vi "AlliGator Script Sequential ROIs Time-Gated Data Series NLSF Analysis.vi"(4 "AlliGator Data Series Type":T10, 8 "Error In":errorcluster, 9 "AlliGator Ctrl Refnums":T1, 10 "Path":path, 11 "Alligator Queue Elements in":T11[](array[typedef])) -> (0 "Error Out":errorcluster, 1 "Message":string, 2 "Time-Series Paths":path[](array[path]), 3 "Alligator Queue Elements out":T11[](array[typedef]))   [LabVIEW 2021, in "AlliGator Scripts.lvlib"]
doc: "Script performing NLSF analysis of a different ROI for each dataset in a series. This is used for instance if the ROI list is representing the successive locations of an object being tracked across the dataset series."
uses:
  AlliGator Scripts.lvlib
  Action Engine/AlliGator Q Element.ctl
  Action Engine/AlliGator Q Event.ctl
  Files/AlliGator Data Series Type.ctl
  GUI/AlliGator Ctrl Refnums.ctl
  GUI/AlliGator Other Ctrl Refnums.ctl
  GUI/AlliGator State Indicator.ctl
  GUI/AlliGator Main Window Tabs.ctl
  GUI/AlliGator Phasor Plot Ctrl Refnums.ctl
  GUI/AlliGator Phasor Graph Ctrl Refnums.ctl
  Phasor/Phasor Calibration Type.ctl
  GUI/AlliGator Dataset Ctrl Refnums.ctl
  Source Image/AlliGator Displayed Image.ctl
  GUI/AlliGator Registered Events Ctrl Refnums.ctl
  GUI/AlliGator Image Histogram Control Refnums.ctl
  Histograms/Linear Histogram Options.ctl
  Histograms/Histogram Bin Option.ctl
  Histograms/Histogram Bin Position.ctl
  Decay Fit Parameter Map/AlliGator Decay Fit Map Control Refnums.ctl
  Fits/IRF(X)PSED/Decay Fit Parameters & Derived Quantities List v2.ctl
  Parameter Map/AlliGator Parameter Map Control Refnums.ctl
  Globals, Variables, Constants/AlliGator Variables List.ctl
  Action Engine/Alligator Elements Order in Action Stack.ctl
  Settings/AlliGator Settings List.ctl
  Fits/Decay Convolution/Decay Model.ctl
  Fits/Residual Type.ctl
  Fits/Non-linear Fitting Method v2.ctl
  Fits/Fit Calculation Method.ctl
  Fits/Non-linear Fitting Algorithm.ctl
  Graphs/XY Graph/New Plot Information.ctl
  Graphs/Plot Scales.ctl
  Graphs/LabVIEW Plot Interpolation.ctl
  Graphs/Plot Point Style.ctl
  ROIs/AlliGator ROI Manager Actions.ctl
  ROIs/AlliGator ROI Selection Data.ctl
  Graphs/XY Graph/XY Graph Selected Plot Info+Flag.ctl
  Graphs/XY Graph/XY Graph Refnum.ctl
  <vilib>/Utility/miscctls.llb/LVPoint32TypeDef.ctl
  Files/AlliGator FLI Dataset Type.ctl
  Action Engine/AlliGator Add Action Array to Stack.vi
  Action Engine/AlliGator Add Single Action to Stack.vi
  Action Engine/AlliGator Action Engine.lvlib
  Globals, Variables, Constants/AlliGator Globals, Variables & Constants.lvlib
  Decay Analysis/Decay Fit/AlliGator Decay Fit.lvlib
  Settings/AlliGator Settings.lvlib
  Fits/Fits.lvlib
  Strings/Strings.lvlib
  Files/Files.lvlib
  Files/AlliGator Files.lvlib
  Graphs/XY Graph/XY Graph Add-Ons.lvlib
  Graphs/Graphs.lvlib
  Variant/Variant.lvlib
  ROIs/AlliGator ROIs.lvlib
  Fits/IRF(X)PSED/Fit Weights Type v2.ctl
  Fits/IRF(X)PSED/Decay Fit Options v4.ctl
  Source Image/AlliGator Source Image.lvlib
  GUI/AlliGator GUI.lvlib
  Phasor/Phasor.lvlib
  Histograms/Histogram Window.lvlib
  Decay Fit Parameter Map/AlliGator Decay Fit Parameter Map.lvlib
  Parameter Map/AlliGator Parameter Map.lvlib
panel:
  out "# Time Points":i32
  # "see the AlliGator License on the block diagram (Ctrl+E or Window:Show Block Diagram)"
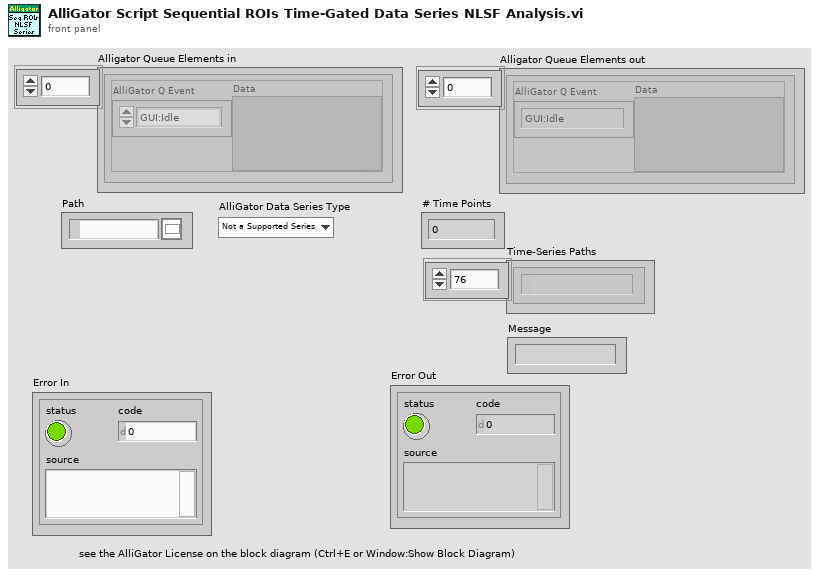
[diagram p1: front panel]
types:
  T1 = typedef "AlliGator GUI.lvlib/AlliGator Ctrl Refnums.ctl" = cluster{"Other AlliGator Ctrl Refnums":T2, "Phasor Plot Ctrl Refnums":T3, "Phasor Graph Ctrl Refnums":T4, "Dataset Control Refnums":T5, "Registered Events Ctrl Refnums":T6, "Image Histogram Ctrl Refnums":T7, "Decay Fit Map Ctrl Refnums":T8, "Parameter Map Ctrl Refnums":T9}
  T2 = typedef "AlliGator GUI.lvlib/AlliGator Other Ctrl Refnums.ctl" = cluster{"State Indicators":refnum<vi>, " Progress Bar":refnum<vi>, "Decay Graph Active":refnum<vi>, "Decay Statistics Bin":refnum<vi>, "Time Step":refnum<vi>, "Use File Timestamp":refnum<vi>, "Tab Control":refnum<vi>, "CPU":refnum<vi>, "Abort Fit":refnum<vi>, "Dataset File/Folder Path":refnum<vi>, "Abort ROI Creation":refnum<vi>, "Event LED":refnum<vi>, "Dataset File/Folder Path 2":refnum<vi>, "Dataset File/Folder Path 3":refnum<vi>, "Dataset File/Folder Path 4":refnum<vi>, "Dataset File/Folder Path 5":refnum<vi>, "Dataset File/Folder Path 6":refnum<vi>, "Dataset File/Folder Path 7":refnum<vi>, "Dataset File/Folder Path 8":refnum<vi>, "Dataset File/Folder Path 9":refnum<vi>, "Dataset File/Folder Path 10":refnum<vi>, "Dataset File/Folder Path 11":refnum<vi>}
  T3 = typedef "AlliGator GUI.lvlib/AlliGator Phasor Plot Ctrl Refnums.ctl" = cluster{"Phasor Ratio":refnum<vi>, "Modulus Lifetime":refnum<vi>, "Phasor at cursor (m, phi)":refnum<vi>, "Phase Lifetime":refnum<vi>, "Phasor at cursor (g, s)":refnum<vi>, "Phasor Plor Average Lifetime":refnum<vi>, "Phasor Plot Active":refnum<vi>, "Save Phasor Plot":refnum<vi>, "Image Overlay Color":refnum<vi>, "Phasor Plot Color Scale":refnum<vi>, "Reference 1 Button":refnum<vi>, "Reference 2 Button":refnum<vi>, "True Phasor Plot Value":refnum<vi>}
  T4 = typedef "AlliGator GUI.lvlib/AlliGator Phasor Graph Ctrl Refnums.ctl" = cluster{"Phasor Ratio":refnum<vi>, "Modulus Lifetime":refnum<vi>, "Phasor at cursor (m, phi)":refnum<vi>, "Phase Lifetime":refnum<vi>, "Phasor at cursor (g, s)":refnum<vi>, "Phasor Graph Average Lifetime":refnum<vi>, "Phasor Graph Active":refnum<vi>, "Save Phasor Graph":refnum<vi>, "Phasor Frame Slide":refnum<vi>, "Single Step Phasor":refnum<vi>, "Calibration Type":refnum<vi>, "Show Line":refnum<vi>, "Phase Lifetime 1":refnum<vi>, "Phase Lifetime 2":refnum<vi>, "Phasor Graph Frequency":refnum<vi>, "Phasor Reference 1 Control":refnum<vi>, "Phasor Reference 2 Control":refnum<vi>, "Calibration Lifetime":refnum<vi>, "Phase Lifetime SDV":refnum<vi>, "Average Lifetime SDV":refnum<vi>, "Phasor Ratio SDV":refnum<vi>, "Modulus Lifetime SDV":refnum<vi>}
  T5 = typedef "AlliGator GUI.lvlib/AlliGator Dataset Ctrl Refnums.ctl" = cluster{"Current Data":refnum<vi>, "Gate Image Slide":refnum<vi>, "Time Point Slide":refnum<vi>, "Current Time Stamp":refnum<vi>, "Save Image":refnum<vi>, "Displayed Image":refnum<vi>, "Overlay Mode":refnum<vi>, "Phasor Overlay Color":refnum<vi>, "Image Color Scale":refnum<vi>, "Use ROI as Search Area":refnum<vi>, "Source Image ROI Color":refnum<vi>, "True Pixel Value":refnum<vi>}
  T6 = typedef "AlliGator GUI.lvlib/AlliGator Registered Events Ctrl Refnums.ctl" = cluster{"Time Point Slider":refnum<vi>, "Phasor Plot Display Range":refnum<vi>, "Decay Graph":refnum<vi>, "Decay Statistics Graph":refnum<vi>, "Intensity Time Trace":refnum<vi>, "Phasor Graph":refnum<vi>, "Phasor Ratio Graph":refnum<vi>, "Lifetime Graph":refnum<vi>, "Phasor Plot Display":refnum<vi>, "Source Image Display":refnum<vi>, "Decay Fit Parameter Map Display Range":refnum<vi>, "Decay Fit Parameter Map Display":refnum<vi>, "Parameter Map Display Range":refnum<vi>, "Parameter Map Display":refnum<vi>, "Phasor Plot Display Range":refnum<vi>}
  T7 = typedef "AlliGator GUI.lvlib/AlliGator Image Histogram Control Refnums.ctl" = cluster{"Image Histogram":refnum<vi>, "Image Histogram Options":refnum<vi>, "Image Histogram Active":refnum<vi>, "Image Histogram Upper Percentile":refnum<vi>, "Image Histogram Lower Percentile":refnum<vi>, "Auto-Adjust Contrast":refnum<vi>}
  T8 = typedef "AlliGator Decay Fit Parameter Map.lvlib/AlliGator Decay Fit Map Control Refnums.ctl" = cluster{"Decay Fit Parameter Map Color Scale":refnum<vi>, "Decay Fit Parameter":refnum<vi>, "Max Parameter":refnum<vi>, "Min Parameter":refnum<vi>, "Decay Fit Parameter Map Display":refnum<vi>, "Decay Fit Parameter Map Display Range":refnum<vi>, "Decay Parameter Map X":refnum<vi>, "Decay Parameter Map Y":refnum<vi>, "Decay Parameter Map Value":refnum<vi>}
  T9 = typedef "AlliGator Parameter Map.lvlib/AlliGator Parameter Map Control Refnums.ctl" = cluster{"Parameter Map Color Scale":refnum<vi>, "Map Parameter":refnum<vi>, "Max Parameter":refnum<vi>, "Min Parameter":refnum<vi>, "Parameter Map Display":refnum<vi>, "Parameter Map Display Range":refnum<vi>, "Parameter Map Set":refnum<vi>, "Parameter Map X":refnum<vi>, "Parameter Map Y":refnum<vi>, "Parameter Map Value":refnum<vi>}
  T10 = typedef "AlliGator Files.lvlib/AlliGator Data Series Type.ctl" = enum16{"Not a Supported Series", "Gate Images Folder Series", "SwissSPAD 2 Dataset Series", "B&H FLI Dataset Series", "PicoQuant PTU FLI Dataset Series", "PicoQuant BIN FLI Dataset Series", "Piccolo hist BIN FLI Dataset Series", "HDF5 FLI Dataset Series"}
  T11 = typedef "AlliGator Action Engine.lvlib/AlliGator Q Element.ctl" = cluster{"AlliGator Q Event":T12, "Data":variant}
  T12 = typedef "AlliGator Action Engine.lvlib/AlliGator Q Event.ctl" = enum16{"---- Files ----", "Files:Set Batch Export Files To Save", "Files:Set Dataset Loading & Pre-processing Options", "Files:Check #Frames in Dataset", "Files:Increment Frame Index", "Files:Open Mask Image", "Files:Open White Light Image", "Files:Open Single Dataset", "Files:New Folder of Folders Selected", "Files:Load File (all Types)_Scriptable", "Files:Move Flattened Series to Folders Series", "Files:Select Folder", "Files:Load FLI Dataset", "Files:Load Swiss SPAD 1 Dataset", "Files:Load Swiss SPAD 2 Dataset", "Files:Load .sdt FLI Dataset", "Files:Load .ptu FLI Dataset", "Files:Load .bin FLI Dataset", "Files:Load Single Gate Image Folder", "Files:Load I/m/phi Dataset (deprecated)", "Files:Load Single Image", "Files:Subtract Background File", "Files:Export FLI Dataset", "Files:Load HDF5 FLI Dataset", "Files:Set Destination File Path", "Files:Save Mask Image", "Files:Batch Conversion", "Files:New Folder Selected", "Files:Close FLI Dataset", "Files:Close FLI Dataset Series", "Files:Close White Light Image", "Files:Close Mask Image", "---- FLI Dataset ----", "FLI Dataset:Channel Arithmetic", "FLI Dataset:Export Average Lifetime Map as ASCII", "FLI Dataset:Export User-Defined Quantity Map as ASCII", "FLI Dataset:Python Function FLI Dataset Event", "FLI Dataset:ROI Analysis", "FLI Dataset:Tilted Logistic Square Gated IRF Characteristics Map", "FLI Dataset:Logistic Square Gated IRF Characteristics Map", "FLI Dataset:Square Gated IRF Characteristics Map", "FLI Dataset:Multi-ROI Single-Pixel Phasor Analysis", "FLI Dataset:Multi-ROI Single-Pixel NLSF Analysis", "FLI Dataset:All ROIs IRF Extraction", "FLI Dataset:All ROIs Decay Fit Non-Interactive (Fast + Individual IRF)", "FLI Dataset:All ROIs Phasor Analysis", "FLI Dataset:All ROIs Decay Fit", "FLI Dataset:Fluorescence Decay Statistics", "FLI Dataset:Update Decay Statistics Graph", "FLI Dataset:Get Decay from ROI", "FLI Dataset:All ROIs Average Lifetimes", "FLI Dataset:Save/Load Local IRFs", "FLI Dataset:Clear Local IRFs", "FLI Dataset:Phasor Calibration Maps (# Gates Series) Script", "FLI Dataset:Calibrated Phasor Map Series", "---- FLI Dataset Series ----", "FLI Dataset Series:Sum All Datasets in Series", "FLI Dataset Series:Add Dataset to Accumulated Dataset", "FLI Dataset Series:Display Accumulated Dataset", "FLI Dataset Series:Clear Dataset Series Sum", "FLI Dataset Series:Time-Series Analysis (NLSF)", "FLI Dataset Series:Time-Series Analysis (Phasor)", "---- Image ----", "Image:Update Image Profile Plots", "Image:Image Histogram Cursor Move", "Image:Image Histogram", "Image:Image Contrast", "Image:Set Image Histogram Cursor Move Flag", "Image:Clear Image Overlay", "Image:Use ROI as Search Area", "Image:Set ROI Diameter", "Image:Save Image Data as TIFF", "Image:Save Displayed Image with Overlay", "Image:Save Image Overlay Only", "Image:Save Image as Hot Pixel Mask", "Image:Change Source Image Color Palette", "Image:Copy Image to Clipboard", "Image:Source Image ROI Selection", "Image:Delete All ROIs", "Image:Delete All Unselected ROIs", "Image:Delete ROI", "Image:Merge All ROIs", "Image:Store ROI", "Image:Source Image ROI Storage", "Image:Export ROI Description to Notebook", "Image:Save ROI", "Image:Load ROI", "Image:Paste ROI Definition", "Image:Clear ROI", "Image:Identify ROIs in Mask Image", "Image:Create Complementary ROI", "Image:Create Contour ROI", "Image:Create ROI(s) from Pixels with Peak above Min_Scriptable", "Image:Create ROI(s) from Pixels with Intensity above Min_Scriptable", "Image:Compute ROI Statistics", "Image:Delete ROI(s) based on ROI Characteristics", "Image:Create ROI Grid", "Image:ROI to Individual Pixel ROIs", "Image:Python Function Source Image Event", "Image:Show Phasor Calibration Map ROI Centers", "Image:Convert ROI to Mask Image", "Image:Mouse Move", "Image:Mouse Up", "Image:Set Source Image Mouse Move Flag", "Image:Add Scale Bar Overlay", "Image:Delete Existing ROIs Option", "Image:Overlay ROI Median", "Image:Check Current ROI", "Image:Update True Pixel Value", "---- Decay ----", "Decay:Clear IRF/Reference Plot", "Decay:Add Decay to Graph", "Decay:Smoothen Plot", "Decay:Smoothen Plot Tail", "Decay:Average Selected Plots", "Decay:Extract IRF", "Decay:Optimal IRF Extraction", "Decay:Threshold IRF", "Decay:Fit to Model IRF", "Decay:Fit IRF to Square Gate", "Decay:Fit IRF to Logistic Square Gate", "Decay:Fit IRF to Tilted Logistic Square Gate", "Decay:Create Bounding Cursors Set", "Decay:Export Bounding Cursors Definition to Notebook", "Decay:Denoise Plot", "Decay:Compute Cumulative Function", "Decay:Use as Reference Decay", "Decay:Show Reference Decay/IRF", "Decay:Extrapolate Decay", "Decay:Create Head & Tail Bounding Cursors", "Decay:Store Cursor-defined Head & Tail Fractions", "Decay:Rebin Plot", "Decay:1-Normalize Decay", "Decay:[0-1]-Normalize Plot", "Decay:Straighten Decay", "Decay:Shift Decay", "Decay:Fold Decay", "Decay:Fit Decay", "Decay:Global Fit of Selected Decays", "Decay:Post Global Fit Script", "Decay:Add Global Fit Parameters to Graph", "Decay:Add Decay Parameter(s) to Plot (Graph)", "Decay:Export Decay to Phasor Graph", "Decay:Compute Average Lifetime", "Decay:Plot Convolution", "Decay:Graph Tip Strip Update", "---- Decay Statistics ----", "Decay Statistics:Tip Strip Update", "---- Intensity Time Trace ----", "Intensity Time Trace:Use File Timestamp", "Intensity Time Trace:Load Intensity Corrections File", "Intensity Time Trace:Clear Intensity Corrections File", "Intensity Time Trace:Tip Strip Update", "---- Phasor Plot ----", "Phasor Plot:Build Phasor Plot", "Phasor Plot:Change Phasor Plot Color Palette", "Phasor Plot:Adjust Phasor Plot Display Range", "Phasor Plot:Highlight Image ROI in Phasor Plot", "Phasor Plot:Save Phasor Plot Image with Overlay", "Phasor Plot:Export Complex Phasor Map", "Phasor Plot:Export Phasor Ratio Map", "Phasor Plot:Export Average Lifetime Map", "Phasor Plot:Compute Phase Lifetime Histogram", "Phasor Plot:Compute Phasor Ratio Histogram", "Phasor Plot:Compute Phase Lifetime vs Intensity Scatter Plot", "Phasor Plot:Weber 2-Component Decomposition", "Phasor Plot:Update Phasor Color Map Vertices", "Phasor Plot:Clear Phasor Overlay", "Phasor Plot:Use Segment Extremities as References", "Phasor Plot:Use UC/Segment Intersections as References", "Phasor Plot:Use UC/Principal Axis Intersections as References", "Phasor Plot:Use UC/Linear Fit Intersections as References", "Phasor Plot:Update Phasor Plot Reference", "Phasor Plot:Show Local Phasor Info in Phasor Plot", "Phasor Plot:Update Phasor Plot State", "Phasor Plot:Phasor Plot ROI Storage", "Phasor Plot:Phasor Plot ROI Selection", "Phasor Plot:Python Function Phasor Plot Event", "Phasor Plot:Overlay Phasor ROI, Ratio or Map in Source Image", "Phasor Plot:Compute Decay of Selected Phasors", "Phasor Plot:Phasor at Image Pixel", "Phasor Plot:Mouse Move", "Phasor Plot:Mouse Up", "Phasor Plot:Display Range Mouse Move", "Phasor Plot:Set Mouse Move Flag", "Phasor Plot:Update True Phasor Plot Value", "---- Phasor Graph ----", "Phasor Graph:Get Phasor Value", "Phasor Graph:Create New Phasor Plot Dialog", "Phasor Graph:Update Last Phasor Value", "Phasor Graph:Update Phasor (m, phi)", "Phasor Graph:Remove Single Phasor from Plot", "Phasor Graph:Add Single Phasor to Plot", "Phasor Graph:Remove Phasor Plot", "Phasor Graph:Remove Selected Phasor Plots", "Phasor Graph:Clear Phasor Data", "Phasor Graph:Clear Phasor Graph", "Phasor Graph:Cursor Move", "Phasor Graph:Draw Cursor Connecting Line", "Phasor Graph:Clear Cursor Connecting Line", "Phasor Graph:Find UC Intersection", "Phasor Graph:Use UC/Cursor-Defined Line Intersections", "Phasor Graph:Use Selected Plots Fitted Line/UC Intersections", "Phasor Graph:Use Selected Plots Principal Axis/UC Intersections", "Phasor Graph:Show Single Phasor", "Phasor Graph:Save Single Phasor Plot", "Phasor Graph:Save All Phasor Plots", "Phasor Graph:Load Phasor Plot(s)", "Phasor Graph:Phasor Multiplication", "Phasor Graph:Compute Average Phasor", "Phasor Graph:Compute Multiple Average Phasors (Selected Plots)", "Phasor Graph:Export Single Phasor Plot Phase Lifetimes", "Phasor Graph:Parameter 2 vs Parameter 1 Scatter Plot", "Phasor Graph:Use Cursor n Location", "Phasor Graph:Set Reference n to Current Phase Lifetime Value", "Phasor Graph:Set Reference n to Lifetime Value", "Phasor Graph:Set Cursor n Location", "Phasor Graph:Save Phasor Graph Image", "Phasor Graph:Update SEPL Plot", "Phasor Graph:Export Single Phasor Plot Data", "Phasor Graph:Export Selected Phasor Plots Data", "Phasor Graph:Python Function Phasor Graph Event", "Phasor Graph:Tip Strip Update", "---- Calibration ----", "Calibration:Set Calibration Type", "Calibration:Load/Save Phasor Calibration", "Calibration:Load/Save Phasor Calibration Series", "Calibration:Load/Save Phasor Calibration Map", "Calibration:Use as Calibration", "Calibration:Compute Optimal Calibration from Phasor References", "Calibration:Clear Phasor Calibration", "Calibration:Single Phasor Calibration Information", "Calibration:Use as Calibration Series", "Calibration:Use as Calibration Map", "Calibration:Clear Calibration Series", "Calibration:Phasor Calibration Series Information", "Calibration:Clear Calibration Map", "Calibration:Phasor Calibration Map Information", "Calibration:Apply Phasor Calibration", "Calibration:Update Single Plot Calibration", "Calibration:Update Multiple Plots Calibration", "Calibration:Clear Single Plot Calibration", "Calibration:Clear All Plots Calibrations", "Calibration:Clear Plot(s) Calibration(s)?", "---- Phasor Ratio ----", "Phasor Ratio:Clear Reference n", "Phasor Ratio:Toggle Selected Plot(s)  Lock to Reference 1", "Phasor Ratio:Use as Reference n", "Phasor Ratio:Send Reference n to Notebook", "Phasor Ratio:Toggle Selected Plot(s)  Lock to Reference 2", "Phasor Ratio:Compute Phasor Ratio at Mouse Location", "Phasor Ratio:Compute Phasor Plot's Average Phasor Ratio", "Phasor Ratio:Compute Time-Series Phasor Ratios", "Phasor Ratio:Fit Line to Phasor Ratio Plot", "Phasor Ratio:Save References", "Phasor Ratio:Load References", "Phasor Ratio:Update Phasor Reference 1", "Phasor Ratio:Update Phasor Reference 2", "Phasor Ratio:Move Cursor n to Reference n", "Phasor Ratio:Use as Phasor Reference 1 Lifetime", "Phasor Ratio:Use as Phasor Reference 2 Lifetime", "Phasor Ratio:Export Phasor Ratio Map as ASCII", "Phasor Ratio:Tip Strip Update", "---- Lifetime & Other Parameters Graph ----", "Lifetime:Compute Sliced Mean, SDV and CV Plots", "Lifetime:Plot Decay Shifts", "Lifetime:Plot Histogram", "---- Decay Fit Parameter Map ----", "Decay Fit Parameter Map:Export ROI NLSF Data as ASCII", "Decay Fit Parameter Map:Set Decay Fit Parameter Map Selection", "Decay Fit Parameter Map:Build Decay Fit Parameter Map", "Decay Fit Parameter Map:Change Decay Fit Parameter Map Color Palette", "Decay Fit Parameter Map:Export Decay Fit Parameter Map Data as ASCII", "Decay Fit Parameter Map:Export All Decay Fit Parameter Maps Data as ASCII", "Decay Fit Parameter Map:Selected Parameter Scatterplot", "Decay Fit Parameter Map:Parameter 2 vs Parameter 1 Scatterplot", "Decay Fit Parameter Map:Save Decay Fit Parameter Map Image", "Decay Fit Parameter Map:Save-Load IRFs & Fit Data", "Decay Fit Parameter Map:Update Local Decay Plots", "Decay Fit Parameter Map:Python Function Decay Fit Parameters Map Event", "Decay Fit Parameter Map:Overlay Decay Fit Parameter Map in Source Image", "Decay Fit Parameter Map:Selected Parameter vs Intensity Scatterplot", "Decay Fit Parameter Map:Mouse Up", "Decay Fit Parameter Map:Mouse Move", "Decay Fit Parameter Map:Display Range Mouse Move", "Decay Fit Parameter Map:Change Map Resolution", "Decay Fit Parameter Map:Variance Significance Maps", "Decay Fit Parameter Map:Fit Result Constraints Window", "---- Parameter Map ----", "Parameter Map:Export ROI Parameters Data as ASCII", "Parameter Map:Delete Parameter Map Set", "Parameter Map:Update Parameter List", "Parameter Map:Build Parameter Map", "Parameter Map:Change Parameter Map Color Palette", "Parameter Map:Export Parameter Map Data as ASCII", "Parameter Map:Export All Parameter Maps Data as ASCII", "Parameter Map:Selected Parameter Scatterplot", "Parameter Map:Parameter 2 vs Parameter 1 Scatterplot", "Parameter Map:Selected Parameter vs Intensity Scatterplot", "Parameter Map:Save Parameter Map Image", "Parameter Map:Save-Load IRFs & Parameter Maps (TODO)", "Parameter Map:Set Parameter Map Selection", "Parameter Map:Python Function Parameter Map Event", "Parameter Map:Overlay Parameter Map in Source Image", "Parameter Map:Update Local Decay Plots", "Parameter Map:Mouse Up", "Parameter Map:Mouse Move", "Parameter Map:Display Range Mouse Move", "---- Generic Graph ----", "Generic Graph:Generic XY Graph Event", "Generic Graph:Python Function XY Graph Event", "Generic Graph:New Plot", "Generic Graph:Save Plot", "Generic Graph:XY Plot Histogram", "Generic Graph:Set XY Graph Plot Name", "Generic Graph:Set Last Cursor Style", "Generic Graph:Tip Strip Update", "---- GUI ----", "GUI:Start Script", "GUI:Type of Displayed Image Changed", "GUI:Gate Image Slide Changed", "GUI:Show Busy Icon", "GUI:Show Busy Icon & Abort Button", "GUI:Hide Busy Icon", "GUI:Hide Busy Icon & Abort Button", "GUI:Abort", "GUI:End Script", "GUI:Start Timing", "GUI:End Timing", "GUI:Set State Indicator", "GUI:Send Parameters JSON Strings to Clipboard", "GUI:Set Gate Step", "GUI:Idle", "GUI:Initialization", "GUI:Quit", "GUI:Increment Dataset Index", "GUI:Set Dataset Index to -1", "GUI:Time Series Slider Moved", "GUI:Time Series Slider Changed", "GUI:Toggle Playback or Loop", "GUI:Playback Script", "GUI:Set Phasor Frequency", "GUI:Open Window", "GUI:Start Test Script", "GUI:End Test Script", "GUI:Set Verbose Mode", "GUI:Set Verbose Settings Mode", "DEBUG"}
  T13 = typedef "AlliGator Globals, Variables & Constants.lvlib/AlliGator Variables List.ctl" = enum16{"---- GUI ----", "GUI:Initialization Status", "GUI:State Indicators Refnum", "GUI:Original AlliGator Menu Items", "GUI:Current Action Loop State", "GUI:Script in progress", "GUI:Playback", "GUI:Loop Playback", "GUI:Search ROI Used", "GUI:Search ROI", "Decay Graph Max Legend Size", "Intensity Graph Max Legend Size", "Decay Statistics Graph Max Legend Size", "Phasor Graph Max Legend Size", "Phasor Ratio Graph Max Legend Size", "Lifetime Graph Max Legend Size", "---- Files ----", "Files:Export Dataset Frames as Individual Files", "Files:Show Batch Export Help Balloons", "Files:Frames in Dataset", "Files:ptu File Frame Start Indices", "Files:Current Frame in Dataset", "Files:Current Frame Timestamp", "Files:Dataset Loaded", "Files:Dataset Metadata", "Files:Dataset Channel", "Files:Dataset Data Description", "Files:Background Dataset Metadata", "Files:Background Dataset Channel", "Files:Background Dataset Data Description", "Files:Background File Subtraction", "Files:Background File Path", "Files:Background File Pile-up Correction", "Files:Background File Pixel Well Capacity", "Files:Background File Scaling Factor", "Files:Current Dataset Load Settings", "Files:Dataset Path", "Files:ICCD-specific Information", "Files:Macrotime Gate Separation", "------ Python Plugins ------", "Python Plugins:Information", "Python Plugins:Python Session", "Python Plugins:Valid Python Session?", "---- Source Image ----", "Source Image:ROIs", "Source Image:Current ROI", "Source Image:ROI Event Refnum", "X_Source Image:Display Range", "X_Source Image:Palette Information", "X_Source Image:Type of Displayed Image", "X_Time Gate Slider", "Source Image:Palette List", "Source Image:Scale", "Source Image:ROI Overlay Color", "Source Image:Overlay to Erase", "Source Image:Is Displayed Image Accumulated", "Source Image:White Light Image Modified", "Source Image:Mask Image Modified", "---- Image Profile Window ----", "Image Profile:Window Event Refnum", "Image Profile:IntensityType", "Image Profile:Intensity Average Type", "Image Profile:Intensity-weighted SDV", "Image Profile:Box Profile Type", "Image Profile:Window Open", "Image Profile:Plotted Fit Parameter", "------ Phasor Graph -------", "Phasor Graph:Show Line", "---- Phasor Plot ---", "Phasor Plot:Parameters Changed", "Phasor Plot:FLI Dataset Modified since last Calculation", "Phasor Harmonics Data", "Selected Phasor Harmonics", "Phasor Harmonic Manager Event Refnum", "Phasor Plot:ROIs", "Phasor Plot:Current ROI", "Phasor Plot:ROI Event Refnum", "Phasor Plot:Image Reference Points", "Phasor Plot:Computed", "Phasor Plot:Palette Information", "Phasor Plot:Palette List", "Phasor Plot:Phasor Ratio Palette Information", "Phasor Plot:Phasor Ratio Palette List", "Phasor Plot:Image Scale", "Phasor Plot:Image Overlay to Erase", "Phasor Plot:Image Elements to Update", "Phasor Plot:Current Calculation Parameters", "Phasor Plot:Current Calibration Options", "Phasor Plot:Reset Cumulated Phasor Plot", "Phasor Plot:Reference 1", "Phasor Plot:Lifetime Reference 1", "Phasor Plot:Reference 1 Frequency", "Phasor Plot:Reference 2", "Phasor Plot:Lifetime Reference 2", "Phasor Plot:Reference 2 Frequency", "---- Decay Analysis ----", "Number of Selected Decays to Fit", "LS Fit Results", "LAR Fit Results", "BS Fit Results", "Last Decay Max - Min", "Best Fit Parameters", "Best Fit Parameter Names", "Actual Size X", "Actual Size Y", "Binning X", "Binning Y", "Actual # Gates", "Dataset Number", "Gates to...", "Gates Skipped", "Gates to keep", "Gate Step", "Gate Separation", "Reversed Gates", "Pile-up Correction", "Pixel Well Capacity", "Background Subtracted", "Background Subtraction Method", "Background Definition Range", "Background File (deprecated)", "Number of Dataset Accumulated", "Array of Accumulated Dataset Paths", "Do Averaged Datasets", "Destination File Path", "Process Plot Target", "Use 1/D as Phasor Frequency", "---- Decay Fit Parameter Map -----", "Decay Fit Parameter Map:Palette Information", "Decay Fit Parameter Map:Palette List", "Decay Fit Parameter Map:X Resolution", "Decay Fit Parameter Map:Y Resolution", "Decay Fit Parameter Map:Use Decay Fit Result Constraints", "Decay Fit Parameter Map:Decay Fit Result Constraints", "Decay Fit Parameter Map:Decay Fit Result Constraints Applied", "---- Parameter Map ----", "Parameter Map:Palette Information", "Parameter Map:Palette List", "------- Local Decay Window ---------", "Local Decay Graph Window:Event Refnum", "Local Decay Graph Window:Use normalized IRF for convolution", "----- Miscellaneous ----", "Misc:Skippable Dialog Windows Status"}
  T14 = enum16{"Start Script", "Load & Analyze Data", "End Script"}
  T15 = typedef "AlliGator ROIs.lvlib/AlliGator ROI Selection Data.ctl" = cluster{"Action":T16, "ID":i32}
  T16 = typedef "AlliGator ROIs.lvlib/AlliGator ROI Manager Actions.ctl" = enum16{"Undefined", "Delete Current ROI", "Delete All Unselected ROIs", "Delete Multiple ROIs", "Delete All ROIs", "Swap ROIs", "Insert ROI", "Update Current ROI Descriptor", "Rename Current ROI", "Store New ROI", "Store Multiple ROIs", "Select Next ROI", "Select Previous ROI", "Find Selected ROI", "Show All ROIs", "Update ROI Manager Window", "Merge All ROIs", "Unmerge ROI", "Set Selected ROI by ID"}
  T17 = typedef "XY Graph Add-Ons.lvlib/New Plot Information.ctl" = cluster{"Multiplot XY Graph":refnum<vi>, "Plot Name":string, "Plot Scales":T18, "Plot Interpolation":T19, "Point Style":T20, "Plot Color":u32, "Plot Metadata":variant}
  T18 = typedef "XY Graph Add-Ons.lvlib/Plot Scales.ctl" = cluster{"X Scale":u32, "Y Scale":u32}
  T19 = typedef "Graphs.lvlib/LabVIEW Plot Interpolation.ctl" = enum16{"Point (.)", "Stepwise Right (--.)", "Line + Point (\\. /)", "Stepwise Left (.--)", "Stepwise Centered (-.-)", "Stepwise Vertical (|.|)", "Line (-)", "Use Previous Plot's Style"}
  T20 = typedef "Graphs.lvlib/Plot Point Style.ctl" = enum16{"not defined", "None", "Empty Circle", "Filled Circle", "Thick Circle", "Dotted Circle", "Empty Square", "Filled Square", "Thick Square", "Dotted Square", "Small Filled Square", "Dot", "Cross", "Tiny Cross", "Large X", "Small x", "Diamond", "Small Empty Square"}
  T21 = typedef "Fits.lvlib/Decay Fit Options v4.ctl" = cluster{"Show Fit Residuals":bool, "Fit Model":T22, "Residual Type":T23, "Max Decay Percentile":dbl, "Min Decay Percentile":dbl, "Show Full Decay":bool, "Weights":T24, "Fitting Method":T25, "Compute Parameter Uncertainties":bool, "Periodic Boundaries":bool, "Model Calculation":T26, "Period":dbl[unit], "Termination Criteria":cluster{"Max Iterations":i32, "Max Function Calls":i32, "Max Time":dbl[unit], "Function Tolerance":dbl, "Parameter Tolerance":dbl, "Gradient Tolerance":dbl, "Min Lambda":dbl, "Max Lambda":dbl, "Initial Tick Count":u32}, "Offset Resolution":dbl[unit], "Use Local IRF":bool, "Fitting Algorithm":T27, "Show Confidence Interval ":bool, "Confidence Level":dbl}
  T22 = typedef "Fits.lvlib/Decay Model.ctl" = enum16{"1-Exponential", "2-Exponentials"}
  T23 = typedef "Fits.lvlib/Residual Type.ctl" = enum16{"Standard", "Normalized", "Reduced"}
  T24 = typedef "Fits.lvlib/Fit Weights Type v2.ctl" = enum16{"Unweighted", "1/Variance (Neyman)", "1/Variance (Pearson)", "Best of All"}
  T25 = typedef "Fits.lvlib/Non-linear Fitting Method v2.ctl" = enum16{"Least Square", "Least Absolute Residual", "Bisquare", "MLE", "-", "Best of All"}
  T26 = typedef "Fits.lvlib/Fit Calculation Method.ctl" = enum16{"Simulation", "Convolution", "Integration"}
  T27 = typedef "Fits.lvlib/Non-linear Fitting Algorithm.ctl" = enum16{"Levenberg-Marquardt", "Trust-Region Dogleg"}
  T28 = typedef "AlliGator Settings.lvlib/AlliGator Settings List.ctl" = enum16{"GUI:Visible Settings Tab", "GUI:Last Run Version", "Source Image:Use Image Histogram for Contrast", "Source Image:Low Count Pixels Rejection Options", "Source Image:High Count Pixels Rejection Options", "Source Image:Use Image Brightness", "Source Image:Blend Overlay with Image Background", "Source Image:Use Fixed ROI Diameter", "Source Image:ROI Diameter", "Source Image:ROI Center Color", "Source Image:Peak Threshold", "Source Image:Intensity Threshold", "Source Image:Image Binning Options", "Source Image:Image Smoothing Options", "Source Image:Image Histogram Active", "Source Image:Invert Binary Mask", "Source Image:Hot Pixel Removal", "Source Image:Overlay Analyzed ROI Center", "Source Image:Auto-Adjust Contrast", "Source Image:Histogram Lower Percentile", "Source Image:Histogram Upper Percentile", "Source Image:Save Source Image", "Source Image:Scale Bar Options", "Source Image:Image Resolution (Pixel Size)", "Source Image:Flatfield Correction", "Source Image:Show Dead Left Columns Correction", "Source Image:Dead Left Columns Correction", "Source Image:Image Pre-Processing Operations Order", "Source Image:Overlay ROI Median", "Source Image:Median Overlay Color", "Data Information:Gate Width", "Data Information:Nanotime Gate Separation", "Data Information:Macrotime Gate Separation", "Data Information:Gate Step", "Data Information:# Gates", "Data Information:Gate Image Exposure", "Data Information:Gate Image Integration", "Data Information:Gates to Skip", "Data Information:Gates to Keep", "Data Information:Define Gates to", "Data Information:Channel Name", "Data Information:Available Channel Names", "Data Information:Channel Arithmetic", "Data Information:Background File Subtraction", "Data Information:Background File", "Data Information:Background Scaling Factor", "Data Information:Background Pile-up Correction", "Data Information:Background Pixel Well Capacity", "Data Information:Laser Period", "Data Information:SYNC Period", "Data Information:Pile-up Correction", "Data Information:Pixel Well Capacity", "Data Information:Dataset Scaling Factor", "Fluorescence Decay_Decay Pre-Processing:Reverse Gates", "Fluorescence Decay_Decay Pre-Processing:Verbose Decay Pre-Processing", "Fluorescence Decay_Decay Pre-Processing:Use Decay Pre-Processing", "Fluorescence Decay_Decay Pre-Processing:Background Subtraction", "Fluorescence Decay_Decay Pre-Processing:Background Definition Range", "Fluorescence Decay_Decay Pre-Processing:Baseline Subtraction Method", "Fluorescence Decay_Decay Pre-Processing:Decay Pre-Processing Operations Order", "Fluorescence Decay_Decay Pre-Processing:Smoothing Parameter", "Fluorescence Decay_Decay Pre-Processing:Shift Decay", "Fluorescence Decay_Decay Pre-Processing:Decay Shift Parameters", "Fluorescence Decay_Decay Pre-Processing:Fold Decay", "Fluorescence Decay_Decay Pre-Processing:# Folds", "Fluorescence Decay_Decay Pre-Processing:1-Normalize Decay", "Fluorescence Decay_Decay Pre-Processing:[0-1]-Normalize Decay", "Fluorescence Decay_Decay Pre-Processing:Smoothen Decay", "Fluorescence Decay_Decay Pre-Processing:Extrapolate Decay", "Fluorescence Decay_Decay Pre-Processing:Use Periodicity", "Fluorescence Decay_Decay Pre-Processing:Use Cursors", "Fluorescence Decay_Decay Pre-Processing:Tail Fraction", "Fluorescence Decay_Decay Pre-Processing:Head Fraction", "Fluorescence Decay_Decay Pre-Processing:Additional Points", "Fluorescence Decay_Decay Pre-Processing:Straighten Decay", "Fluorescence Decay_Decay Pre-Processing:Constant Background", "Fluorescence Decay_Decay Pre-Processing:Pixel-Normalize Decay", "Fluorescence Decay_Advanced Analysis:Extract IRF instead of Decay", "Fluorescence Decay_Advanced Analysis:IRF Extraction Options", "Fluorescence Decay_Advanced Analysis:IRF Optimization Options", "Fluorescence Decay_Advanced Analysis:Square Pulse Options", "Fluorescence Decay_Advanced Analysis:IRF Order", "Fluorescence Decay_Advanced Analysis:IRF Time Constants", "Fluorescence Decay_Advanced Analysis:Wavelet Analysis Options", "Fluorescence Decay_Advanced Analysis:Average Lifetime Options", "Fluorescence Decay_Fit Options:Fit Options", "Fluorescence Decay_Fit Options:Use Legacy Fitting Approach", "Fluorescence Decay_Fit Options:Use Data Information Laser Period", "Fluorescence Decay_Fit Parameters:Displayed Fit Parameters", "Fluorescence Decay_Fit Parameters:Fit Parameter Constraints", "Fluorescence Decay_Fit Parameters:Export Tabulated Results", "Fluorescence Decay_Fit Parameters:MLE Baseline Offset Type", "Fluorescence Decay_Fit Parameters:MLE Baseline Offset", "Fluorescence Decay_Fit Parameters:Guess Parameter Names", "Fluorescence Decay_Fit Parameters:Guess Parameter Values", "Fluorescence Decay_Fit Parameters:Guess Parameters Options", "Fluorescence Decay_Fit Parameters:Optimal Offset Selection Criterion", "Fluorescence Decay_Styles:Show Last Decay Only", "Fluorescence Decay_Styles:Decay Graph Color Array", "Fluorescence Decay:Decay Graph Active", "Fluorescence Decay Statistics:Min Peak Value", "Fluorescence Decay Statistics:Reject Low Decay Peak Pixels", "Fluorescence Decay Statistics:Reject High Decay Peak Pixels", "Fluorescence Decay Statistics:Max Peak Value", "Time Traces:Use File Timestamp", "Time Traces:Time Step", "Time Traces:Use Intensity Correction File", "Time Traces:Intensity Correction File", "Phasor Plot:Phasor Plot Smoothing Options", "Phasor Plot:Phasor Plot Size", "Phasor Plot:Phasor Plot Graphics Options", "Phasor Plot:Cumulative Phasor Plot", "Phasor Plot:Use Phasor Brightness", "Phasor Plot:Blend Overlay with Phasor Background", "Phasor Plot:Save Phasor Plot", "Phasor Plot:Show References", "Phasor Plot:Phasor Ratio Decay Range", "Phasor Plot:Exponential Fading", "Phasor Plot:Phasor Ratio Reference Colors", "Phasor Plot:Reference Radius", "Phasor Plot:Show Color Map Vertices", "Phasor Plot:Phasor Plot Active", "Phasor Plot:Phasor Ratio Color Map Type", "Phasor Plot:Phasor Ratio Color Map", "Phasor Plot:Phasor Ratio Display Range", "Phasor Plot:Selected Image ROI(s)", "Phasor Plot:All Image ROIs", "Phasor Plot:Selected Phasor Plot ROI(s)", "Phasor Plot:All Phasor Plot ROIs", "Phasor Plot:Phasor Ratio Color-Coded Quantity", "Phasor Plot:Store Phasor Harmonics", "Phasor Plot:Draw Reference Segment", "Phasor Plot:User-Defined Quantity", "Phasor Plot:Color Scale High Color", "Phasor Plot:Color Scale Low Color", "Phasor Plot:Intensity-weighted Phasor Plot", "Phasor Graph:Phasor Frequency", "Phasor Graph:Phasor Ratio Type", "Phasor Graph:Pixel-level Phasor Computation", "Phasor Graph:Save Phasor Graph", "Phasor Graph:Phasor Graph Active", "Phasor Graph:Phasor SDV Options", "Phasor Graph:Intensity-weighted Phasor Graph", "Phasor Graph:Define Shortest Lifetime as", "Phasor Calibration:Use Backup Calibration if needed", "Phasor Calibration:Backup Calibration Type", "Phasor Calibration:Calibration Type", "Phasor Calibration:Calibration Lifetime", "Phasor Calibration:Calibration Map Algorithm", "Single-Exponential Phasor Locus (SEPL):Gate Parameters", "Single-Exponential Phasor Locus (SEPL):User-defined Gate", "Single-Exponential Phasor Locus (SEPL):User-defined IRF", "Single-Exponential Phasor Locus (SEPL):Phasor Parameters", "Single-Exponential Phasor Locus (SEPL):Decay & IRF Parameters", "Single-Exponential Phasor Locus (SEPL):Display Parameters", "Lifetime Analysis:Decay Analysis Parameters", "Lifetime Analysis:Lifetime Map Active", "Plugins:Python Settings", "Miscellaneous:Verbose Mode", "Miscellaneous:Beep after Script", "Miscellaneous:Saved Image File Format", "Miscellaneous:Exported Gate Image Settings", "Miscellaneous:Include Loading in Timing", "Miscellaneous:Verbose Settings Mode", "Miscellaneous:Histogram Options", "Miscellaneous:Beep on Error", "Miscellaneous:# Logical Processors Used", "Miscellaneous:ROI Description Max Characters", "Miscellaneous:Verbose Error Mode", "Miscellaneous:Transparent Mask Color"}
  T29 = typedef "AlliGator Action Engine.lvlib/Alligator Elements Order in Action Stack.ctl" = enum16{"Enqueue 2 AFTER 1", "Enqueue 2 BEFORE 1"}
  T30 = typedef "XY Graph Add-Ons.lvlib/XY Graph Selected Plot Info+Flag.ctl" = cluster{"Multiplot XY Graph":T31, "Mouse Coordinates":T32, "Plot Index":i32, "Flag":bool}
  T31 = typedef "XY Graph Add-Ons.lvlib/XY Graph Refnum.ctl" = refnum<vi>
  T32 = typedef "LVPoint32TypeDef.ctl" = cluster{"Horizontal":i32, "Vertical":i32}
  T33 = typedef "AlliGator Files.lvlib/AlliGator FLI Dataset Type.ctl" = enum16{"HDF5 FLI Dataset", "Gate Image Folder", ".sdt FLI Dataset (Becker & Hickl)", ".ptu FLI Dataset (PicoQuant)", "SS1 FLI Dataset", "SS2 FLI Dataset", "I/m/phi Dataset", ".bin FLI Dataset (PicoQuant Binned)", ".bin FLI Dataset (Piccolo Binned)", ".mat FLI Dataset"}
  T34 = typedef "AlliGator Displayed Image.ctl" = enum16{"Single Gate", "Sum of All Gates", "Max of All Gates", "Min of All Gates", "-", "White Ligth Image", "Mask Image"}
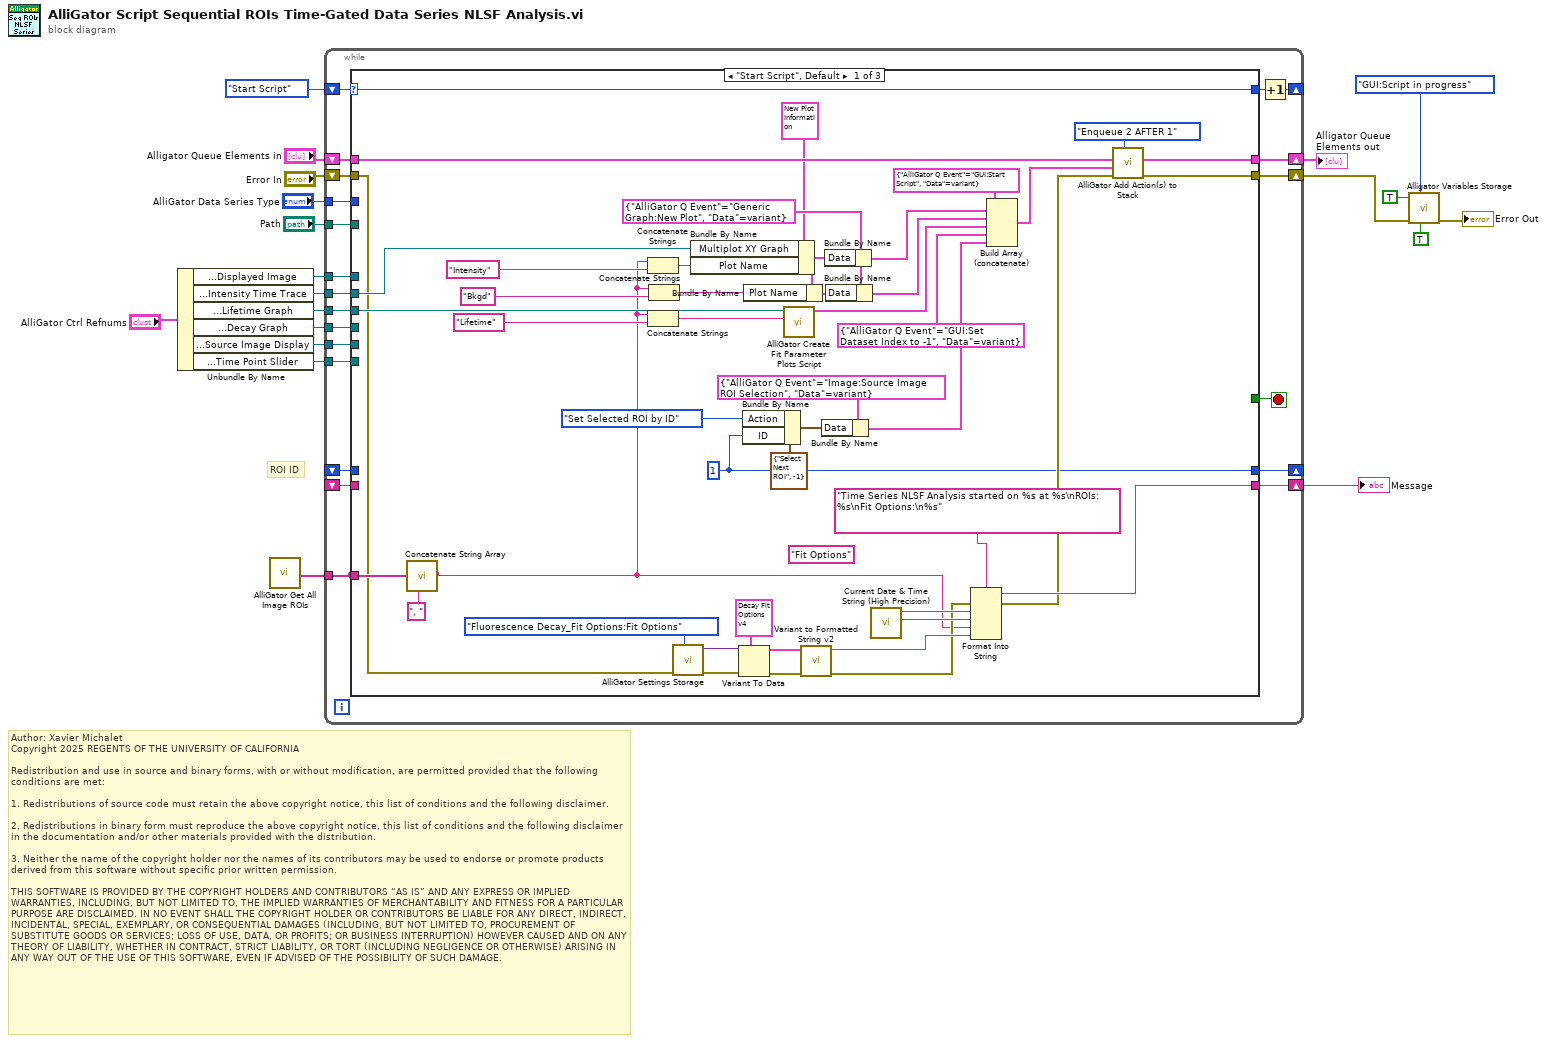
[diagram p0: block diagram]
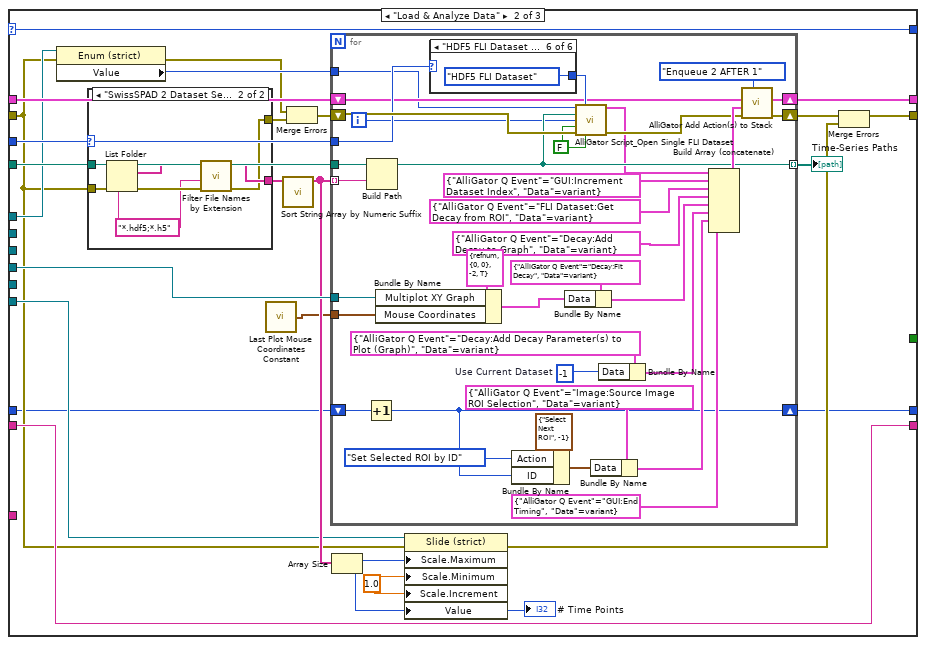
[diagram p2: hidden frame]
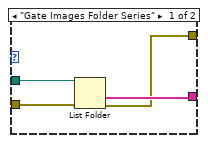
[diagram p3: hidden frame]
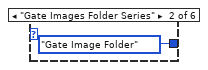
[diagram p5: hidden frame]
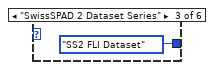
[diagram p6: hidden frame]
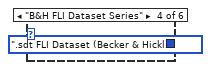
[diagram p7: hidden frame]
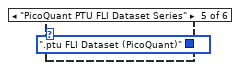
[diagram p8: hidden frame]
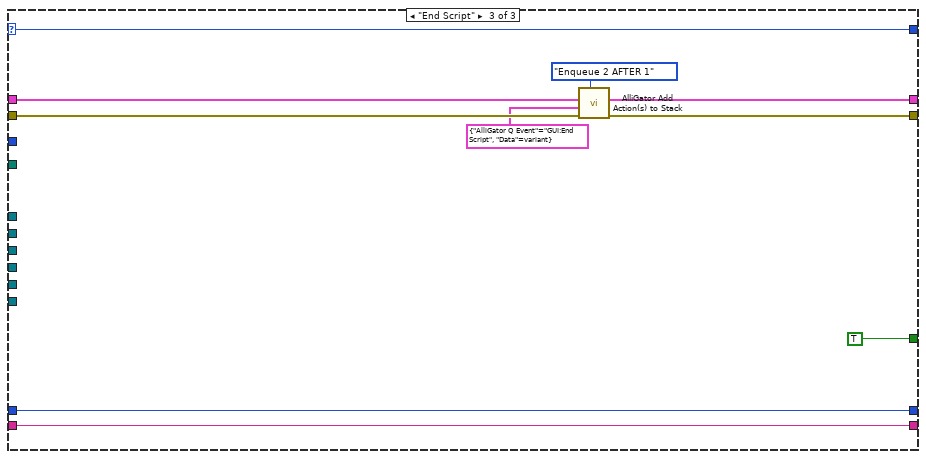
[diagram p9: hidden frame]
diagram:
  # "ROI ID"
  # "Author: Xavier Michalet\nCopyright 2025 REGENTS OF THE UNIVERSITY OF CALIFORNIA\n\nRedistribution and use in source and binary forms, with or without modification, are permitted provided that the following conditions are met:\n\n1. Redistributions of source code must retain the above copyright notice, this list of conditions and the following disclaimer.\n\n2. Redistributions in binary form must reproduce the above copyright notice, this list of conditions and the following disclaimer in the documentation and/or other materials provided with the distribution.\n\n3. Neither the name of the copyright holder nor the names of its contributors may be used to endorse or promote products derived from this software without specific prior written permission.\n\nTHIS SOFTWARE IS PROVIDED BY THE COPYRIGHT HOLDERS AND CONTRIBUTORS “AS IS” AND ANY EXPRESS OR IMPLIED WARRANTIES, INCLUDING, BUT NOT LIMITED TO, THE IMPLIED WARRANTIES OF MERCHANTABILITY AND FITNESS FOR A PARTICULAR PURPOSE ARE DISCLAIMED. IN NO EVENT SHALL THE COPYRIGHT HOLDER OR CONTRIBUTORS BE LIABLE FOR ANY DIRECT, INDIRECT, INCIDENTAL, SPECIAL, EXEMPLARY, OR CONSEQUENTIAL DAMAGES (INCLUDING, BUT NOT LIMITED TO, PROCUREMENT OF SUBSTITUTE GOODS OR SERVICES; LOSS OF USE, DATA, OR PROFITS; OR BUSINESS INTERRUPTION) HOWEVER CAUSED AND ON ANY THEORY OF LIABILITY, WHETHER IN CONTRACT, STRICT LIABILITY, OR TORT (INCLUDING NEGLIGENCE OR OTHERWISE) ARISING IN ANY WAY OUT OF THE USE OF THIS SOFTWARE, EVEN IF ADVISED OF THE POSSIBILITY OF SUCH DAMAGE."
  n1 = Unbundle By Name("AlliGator Ctrl Refnums") -> ("Dataset Control Refnums.Displayed Image"=w2:refnum<vi>, "Registered Events Ctrl Refnums.Intensity Time Trace"=w5:refnum<vi>, "Registered Events Ctrl Refnums.Lifetime Graph"=w10:refnum<vi>, "Registered Events Ctrl Refnums.Decay Graph"=w9:refnum<vi>, "Registered Events Ctrl Refnums.Source Image Display"=w4:refnum<vi>, "Registered Events Ctrl Refnums.Time Point Slider"=w3:refnum<vi>)
  n2 = call "AlliGator Get All Image ROIs.vi"() -> ("ROI Names"=w1:string[])  [unwired: 9 in]
  n3 = while {
    tunnel: "Path" -> [w40]
    shift-right: [w37] -> w15
    shift-left: "Error In" -> [w41]
    shift-right: [w35] -> _
    shift-left: T14."Start Script" -> [w38]
    shift-right: [w33] -> w16
    shift-left: "Alligator Queue Elements in" -> [w39]
    tunnel: w10 -> [w32]
    tunnel: w9 -> [w31]
    tunnel: w1 -> [w30]
    tunnel: [w30] -> _
    tunnel: "AlliGator Data Series Type" -> [w29]
    shift-right: [w28] -> w7
    shift-left: _ -> [w27]
    tunnel: w5 -> [w26]
    tunnel: w4 -> [w25]
    tunnel: w3 -> [w24]
    tunnel: w2 -> [w23]
    shift-right: [w22] -> _
    shift-left: _ -> [w21]
    stop <- w34 stop-if-true
    n4 = case shown="\"Start Script\", Default" w38 {
      selector: w38 -> [w87 w111 w173]
      tunnel: w41 -> [w43 w95 w170]
      tunnel: w40 -> [_ w99 _]
      tunnel: w39 -> [w85 w112 w171]
      tunnel: [w58 w92 w167] -> w37
      tunnel: [w87 w111 w173] -> w36
      tunnel: [_ _ TRUE] -> w34
      tunnel: [w84 w109 w168] -> w33
      tunnel: w32 -> [w71 _ _]
      tunnel: w31 -> [_ w105 _]
      tunnel: w30 -> [w45 _ _]
      tunnel: w29 -> [_ w101 _]
      tunnel: [w57 w102 w166] -> w28
      tunnel: w27 -> [_ w102 w166]
      tunnel: w26 -> [w54 _ _]
      tunnel: w25 -> [_ _ _]
      tunnel: w24 -> [_ w98 _]
      tunnel: w23 -> [_ w97 _]
      tunnel: [w42 w88 w165] -> w22
      tunnel: w21 -> [_ w89 w165]
      frame "Start Script", Default {
        w42 = 1 ("ID")
        (unwired) "Fit Options" ("Label")
        w72 = T11 {"AlliGator Q Event"=enum."Generic Graph:New Plot", "Data"=variant} ("element")
        n5 = call "Concatenate String Array.vi"("Separator (TAB)"=", ", "String Array"=w45) -> ("Formatted String"=w44:string)  [unwired: 9 in]
        n6 = Concatenate Strings(w44, "Intensity" ("Plot Name")) -> (w74:string)
        n7 = Concatenate Strings(w44, "Lifetime" ("Plot Name")) -> (w75:string)
        n8 = Concatenate Strings(w44, "Bkgd" ("Plot Name")) -> (w73:string)
        n9 = call "AlliGator Settings Storage.vi"("AlliGator Settings List"=AlliGator_Settings_List."Fluorescence Decay_Fit Options:Fit Options", "Error In"=w43) -> ("Error Out"=w68:errorcluster, "Variant Data out"=w69:variant)  [unwired: 8 in]
        n10 = Bundle By Name(cluster=T17 {"Multiplot XY Graph"=refnum, "Plot Name"="", "Plot Scales"={"X Scale"=0, "Y Scale"=0}, "Plot Interpolation"=enum."Use Previous Plot's Style", "Point Style"=enum."not defined", "Plot Color"=15781887, "Plot Metadata"=variant} ("New Plot Information"), "Multiplot XY Graph"=w54, "Plot Name"=w74) -> (w81:T17)
        n11 = Variant To Data(error in=w68, type=T21 {"Show Fit Residuals"=TRUE, "Fit Model"=enum."1-Exponential", "Residual Type"=enum."Standard", "Max Decay Percentile"=0.0, "Min Decay Percentile"=0.0, "Show Full Decay"=TRUE, "Weights"=enum."Unweighted", "Fitting Method"=enum."Least Square", "Compute Parameter Uncertainties"=TRUE, "Periodic Boundaries"=TRUE, "Model Calculation"=enum."Simulation", "Period"=1.2500000000000001e-08, "Termination Criteria"={"Max Iterations"=1000, "Max Function Calls"=0, "Max Time"=1000.0, "Function Tolerance"=1e-06, "Parameter Tolerance"=1e-06, "Gradient Tolerance"=0.0, "Min Lambda"=1e-06, "Max Lambda"=1e-06, "Initial Tick Count"=0}, "Offset Resolution"=1.2500000000000001e-08, "Use Local IRF"=TRUE, "Fitting Algorithm"=enum."Levenberg-Marquardt", "Show Confidence Interval "=TRUE, "Confidence Level"=95.0} ("Fit Options"), Variant=w69) -> (data=w60:T21, error out=w67:errorcluster)
        n12 = Bundle By Name(cluster=T15 {"Action"=enum."Select Next ROI", "ID"=-1} ("ROI Selection Data"), "Action"=AlliGator_ROI_Manager_Actions."Set Selected ROI by ID", "ID"=w42) -> (w51:T15)
        n13 = Bundle By Name(cluster=w81, "Plot Name"=w73) -> (w77:T17)
        n14 = call "AlliGator Create Fit Parameter Plots Script.vi"("Current ROI Name"=w75, "XYGraph in"=w71) -> ("AlliGator Script"=w70:T11[])  [unwired: 9 in]
        n15 = call "Variant to Formatted String v2.vi"("error in (no error)"=w67, "Anything"=w60) -> ("error out"=w53:errorcluster, "String"=w66:string)  [unwired: 8 in]
        n16 = Bundle By Name(cluster=T11 {"AlliGator Q Event"=enum."Image:Source Image ROI Selection", "Data"=variant} ("Time-Gated Phasor Q Element"), "Data"=w51) -> (w47:T11)
        n17 = Bundle By Name(cluster=w72, "Data"=w81) -> (w80:T11)
        n18 = Bundle By Name(cluster=w72, "Data"=w77) -> (w78:T11)
        n19 = call "Current Date & Time String (High Precision).vi"() -> ("time string"=w61:string, "date string"=w62:string)  [unwired: 8 in, 2 out]
        n20 = Format Into String(format string="Time Series NLSF Analysis started on %s at %s\nROIs: %s\nFit Options:\n%s" ("initial string"), error in=w53, w62, w61, w44, w66) -> (resulting string=w57:string, error out=w52:errorcluster)  [unwired: 1 in]
        n21 = Build Array (concatenate)(T11 {"AlliGator Q Event"=enum."GUI:Start Script", "Data"=variant} ("element"), w80, w78, w70, T11 {"AlliGator Q Event"=enum."GUI:Set Dataset Index to -1", "Data"=variant} ("element"), w47) -> (w83:T11[])
        n22 = call-poly "AlliGator Add Action(s) to Stack.vi"("Elements Order in Action Stack (Default: 2 BEFORE 1)"=Alligator_Elements_Order_in_Action_Stack."Enqueue 2 AFTER 1", "Error In"=w52, "Alligator Queue Element 2"=w83, "Alligator Queue Element 1"=w85) -> ("Error Out"=w58:errorcluster, "Alligator Queue Element 1 (+ 2)"=w84:T11[])  [unwired: 6 in]
      }
      frame "Load & Analyze Data" {
        w108 = 1.0 ("Scale.Range:Minimum")
        n23 = property class="Enum (strict)"(reference=w97, error in=w95) -> (error out=w93:errorcluster, "Value"=w96:T34)  [unwired: 1 out]
        n24 = case shown="\"SwissSPAD 2 Dataset Series\", Default" w101 {
          tunnel: [w114 w123] -> w103
          tunnel: w99 -> [w116 w122]
          tunnel: w95 -> [w115 w121]
          tunnel: [w113 w118] -> w100
          frame "Gate Images Folder Series" {
            n25 = List Folder(path=w116, error in=w115) -> (folder names=w114:string[], error out=w113:errorcluster)  [unwired: 2 in, 2 out]
          }
          frame "SwissSPAD 2 Dataset Series", Default {
            w119 = "*.hdf5;*.h5" ("patterns")
            n26 = List Folder(path=w122, pattern=w119, error in=w121) -> (filenames=w117:string[], error out=w120:errorcluster)  [unwired: 1 in, 2 out]
            n27 = call "Filter File Names by Extension.vi"("Error In"=w120, "patterns"=w119, "filenames in"=w117) -> ("Error Out"=w118:errorcluster, "filenames out"=w123:string[])  [unwired: 6 in, 1 out]
          }
        }
        n28 = call "Last Plot Mouse Coordinates Constant.vi"() -> ("Selected Plots Mouse Coordinates Equivalent"=w90:T32)
        n29 = call "Sort String Array by Numeric Suffix.vi"("String Array"=w103) -> ("Sorted String Array"=w104:string[])  [unwired: 8 in, 2 out]
        n30 = Merge Errors(w93, w100) -> (w94:errorcluster)
        n31 = for {
          shift-right: [w158] -> w109
          shift-left: w112 -> [w142]
          shift-right: [w156] -> w110
          shift-left: w94 -> [w155]
          tunnel: [w149] -> w106 mode=indexing
          tunnel: w105 -> [w152]
          tunnel: w104 -> [w150] mode=indexing
          tunnel: w99 -> [w151]
          tunnel: w101 -> [w147]
          tunnel: w96 -> [w139]
          tunnel: w90 -> [w132]
          shift-right: [w124] -> w88
          shift-left: w89 -> [w125]
          i -> [w126]
          w128 = -1  # Use Current Dataset
          w138 = FALSE ("Save Image with Overlay")
          n32 = Increment(x=w125) -> (x+1=w124:i32)
          n33 = Build Path(base path=w151, name or relative path=w150) -> (appended path=w149:path)
          n34 = Bundle By Name(cluster=T30 {"Multiplot XY Graph"=refnum, "Mouse Coordinates"={"Horizontal"=0, "Vertical"=0}, "Plot Index"=-2, "Flag"=TRUE} ("Last Plot, Display"), "Multiplot XY Graph"=w152, "Mouse Coordinates"=w132) -> (w130:T30)
          n35 = case shown="\"HDF5 FLI Dataset Series\"" w147 {
            tunnel: [_ AlliGator_FLI_Dataset_Type."Gate Image Folder" ("FLI Dataset Type") AlliGator_FLI_Dataset_Type."SS2 FLI Dataset" ("FLI Dataset Type") AlliGator_FLI_Dataset_Type.".sdt FLI Dataset (Becker & Hickl)" ("FLI Dataset Type") AlliGator_FLI_Dataset_Type.".ptu FLI Dataset (PicoQuant)" ("FLI Dataset Type") AlliGator_FLI_Dataset_Type."HDF5 FLI Dataset" ("FLI Dataset Type")] -> w146
            frame "Not a Supported Series", Default {
            }
            frame "Gate Images Folder Series" {
            }
            frame "SwissSPAD 2 Dataset Series" {
            }
            frame "B&H FLI Dataset Series" {
            }
            frame "PicoQuant PTU FLI Dataset Series" {
            }
            frame "HDF5 FLI Dataset Series" {
            }
          }
          n36 = Bundle By Name(cluster=T15 {"Action"=enum."Select Next ROI", "ID"=-1} ("ROI Selection Data"), "Action"=AlliGator_ROI_Manager_Actions."Set Selected ROI by ID", "ID"=w124) -> (w137:T15)
          n37 = Bundle By Name(cluster=T11 {"AlliGator Q Event"=enum."Decay:Fit Decay", "Data"=variant} ("element"), "Data"=w130) -> (w154:T11)
          n38 = call "AlliGator Script_Open Single FLI Dataset.vi"("Type of Displayed Image"=w139, "FLI Dataset Type"=w146, "File Path"=w149, "Dataset index in Series (0)"=w126, "Save Image with Overlay"=w138, "Error In"=w155, "Save Phasor Plot with Overlay"=w138) -> ("Action List out"=w143:T11[], "Error Out"=w148:errorcluster)  [unwired: 7 in]
          n39 = Bundle By Name(cluster=T11 {"AlliGator Q Event"=enum."Image:Source Image ROI Selection", "Data"=variant} ("Time-Gated Phasor Q Element"), "Data"=w137) -> (w133:T11)
          n40 = Bundle By Name(cluster=T11 {"AlliGator Q Event"=enum."Decay:Add Decay Parameter(s) to Plot (Graph)", "Data"=variant} ("element"), "Data"=w128) -> (w144:T11)
          n41 = Build Array (concatenate)(w143, T11 {"AlliGator Q Event"=enum."GUI:Increment Dataset Index", "Data"=variant} ("element"), T11 {"AlliGator Q Event"=enum."FLI Dataset:Get Decay from ROI", "Data"=variant} ("element"), T11 {"AlliGator Q Event"=enum."Decay:Add Decay to Graph", "Data"=variant} ("element"), w154, w144, w133, T11 {"AlliGator Q Event"=enum."GUI:End Timing", "Data"=variant} ("element")) -> (w157:T11[])
          n42 = call-poly "AlliGator Add Action(s) to Stack.vi"("Elements Order in Action Stack (Default: 2 BEFORE 1)"=Alligator_Elements_Order_in_Action_Stack."Enqueue 2 AFTER 1", "Error In"=w148, "Alligator Queue Element 2"=w157, "Alligator Queue Element 1"=w142) -> ("Error Out"=w156:errorcluster, "Alligator Queue Element 1 (+ 2)"=w158:T11[])  [unwired: 6 in]
        }
        "Time-Series Paths" <- w106
        n43 = Array Size(array=w104) -> (size(s)=w107:i32)
        "# Time Points" <- w107
        n44 = property class="Slide (strict)"(reference=w98, error in=w95, "Scale.Maximum"=w107, "Scale.Minimum"=w108, "Scale.Increment"=w108, "Value"=w107) -> (error out=w91:errorcluster)  [unwired: 1 out]
        n45 = Merge Errors(w110, w91) -> (w92:errorcluster)
      }
      frame "End Script" {
        n46 = call-poly "AlliGator Add Action(s) to Stack.vi"("Elements Order in Action Stack (Default: 2 BEFORE 1)"=Alligator_Elements_Order_in_Action_Stack."Enqueue 2 AFTER 1", "Error In"=w170, "Alligator Atomic Action"=T11 {"AlliGator Q Event"=enum."GUI:End Script", "Data"=variant} ("element"), "Alligator Queue Element 1"=w171) -> ("Error Out"=w167:errorcluster, "Alligator Queue Element 1 (+ 2)"=w168:T11[])  [unwired: 6 in]
      }
    }
    n47 = Increment(x=w36) -> (x+1=w35:T14)
  }
  "Alligator Queue Elements out" <- w16
  "Message" <- w7
  n48 = call "Alligator Variables Storage.vi"("Get(F)/Set"=TRUE, "AlliGator Variable"=AlliGator_Variables_List."GUI:Script in progress" ("Alligator Variable"), "Error In"=w15, "Data in"=TRUE) -> ("Error Out"=→"Error Out":errorcluster)  [unwired: 5 in, 2 out]
